vi "Tosca-Initialize Schedule State.vi"(0 "Tosca":refnum<class "Parameters.lvclass">, 11 "error in (no error)":errorcluster, 12 "Analysis In":T2, 13 "Controls":T1) -> (2 "Blocks":i32, 4 "Tosca out":refnum<class "Parameters.lvclass">, 14 "Analysis Out":T2, 15 "error out":errorcluster)   [LabVIEW 2020]
uses:
  Typedefs/Tosca-Analysis State.ctl
  Typedefs/Tosca-Adaptation State.ctl
  Typedefs/Tosca-Adaptation Track State.ctl
  Typedefs/Tosca-Adaptation History Element.ctl
  Classes/Parameters/Histogram Data.ctl
  Classes/Parameters/Connect.ctl
  Typedefs/Tosca-Control Refs.ctl
  FSM Graph VIs/LV Source/FSM Editor/FSM Editor.xctl
  Classes/Parameters/Parameters.lvclass
  Classes/Parameters/Parameters.lvclass/Parameters.ctl
  Classes/Parameters/Read Schedule.vi
  Classes/Parameters/Read Schedule Mode.vi
  Classes/Parameters/Read Adapt.vi
  Classes/Parameters/Write Adapt.vi
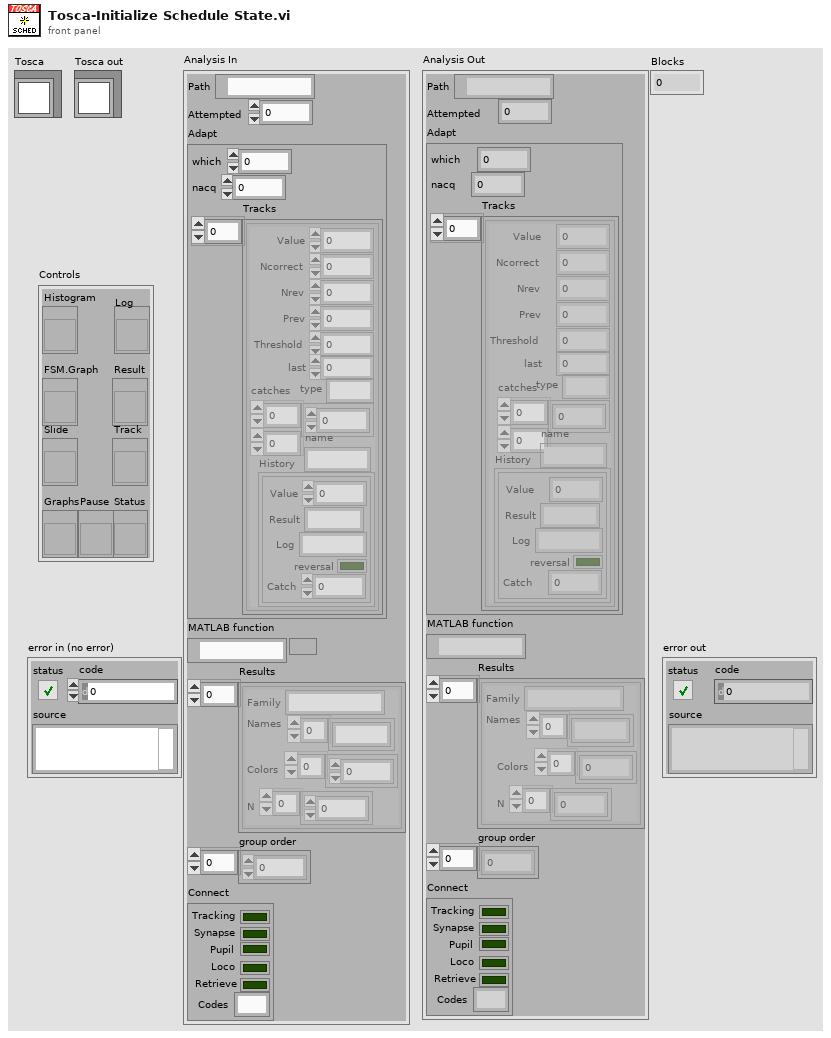
[diagram p1: front panel]
types:
  T1 = typedef "Tosca-Control Refs.ctl" = cluster{"FSM.Graph":refnum<vi>, "Slide":refnum<vi>, "Result":refnum<vi>, "Histogram":refnum<vi>, "Graphs":refnum<vi>, "Track":refnum<vi>, "Log":refnum<vi>, "Status":refnum<vi>, "Pause":refnum<vi>}
  T2 = typedef "Tosca-Analysis State.ctl" = cluster{"Path":path, "Attempted":i32, "Adapt":T3, "MATLAB function":path, "Results":T6[], "group order":i32[], "Connect":T7}
  T3 = typedef "Tosca-Adaptation State.ctl" = cluster{"which":i32, "nacq":i32, "Tracks":T4[]}
  T4 = typedef "Tosca-Adaptation Track State.ctl" = cluster{"Value":dbl, "Ncorrect":i32, "Nrev":i32, "Prev":dbl, "History":T5[], "Threshold":dbl, "last":i32, "type":string, "catches":dbl[][], "name":string}
  T5 = typedef "Tosca-Adaptation History Element.ctl" = cluster{"Value":dbl, "Result":string, "Log":string, "reversal":bool, "Catch":dbl}
  T6 = typedef "Parameters.lvclass/Histogram Data.ctl" = cluster{"Family":string, "Names":string[], "Colors":u32[], "N":i32[]}
  T7 = typedef "Parameters.lvclass/Connect.ctl" = cluster{"Tracking":bool, "Synapse":bool, "Pupil":bool, "Loco":bool, "Retrieve":bool, "Codes":string}
  T8 = typedef "Tosca-Schedule.ctl" = cluster{"Blocks":i32, "order":T9, "balance":bool, "Families":T10[]}
  T9 = typedef "Tosca-Sequence Order.ctl" = enum16{"Sequential", "Alternate", "Randomize", "Random group"}
  T10 = typedef "Tosca-Parameter Family.ctl" = cluster{"Name":string, "Number":i32, "Vars":T11[], "Mask":bool[][], "one each":bool}
  T11 = typedef "Tosca-Parameter Table Element.ctl" = cluster{"state":string, "chan":string, "param":string, "expr":string, "dim":T12, "value":dbl[]}
  T12 = typedef "Tosca-Parameter Dimension.ctl" = enum16{"Ind", "X", "Y"}
  T13 = typedef "Tosca-Schedule Mode.ctl" = enum16{"Seq", "CS+/CS-", "Adapt"}
  T14 = typedef "Tosca-Adapt.ctl" = cluster{"Switch after":i32, "Switch type":enum16{"Trials", "Reversals"}, "Tracks":T15[]}
  T15 = typedef "Tosca-Adaptive Track.ctl" = cluster{"state":string, "chan":string, "param":string, "Start":dbl, "Step":string, "Mode":enum16{"Add", "Multiply"}, "Pcatch":dbl, "Ndown":i32, "Nup":i32, "Nreverse":i32, "Min":dbl, "Max":dbl, "Catch":T16[], "do all catch":bool, "name":string, "Vars":T16[], "compute":T17, "of last":i32, "Step2":string, "after":i32}
  T16 = typedef "Tosca-Simple Variable.ctl" = cluster{"state":string, "chan":string, "param":string, "expr":string}
  T17 = typedef "Tosca-Adapt Threshold Metric.ctl" = enum16{"mean", "median"}
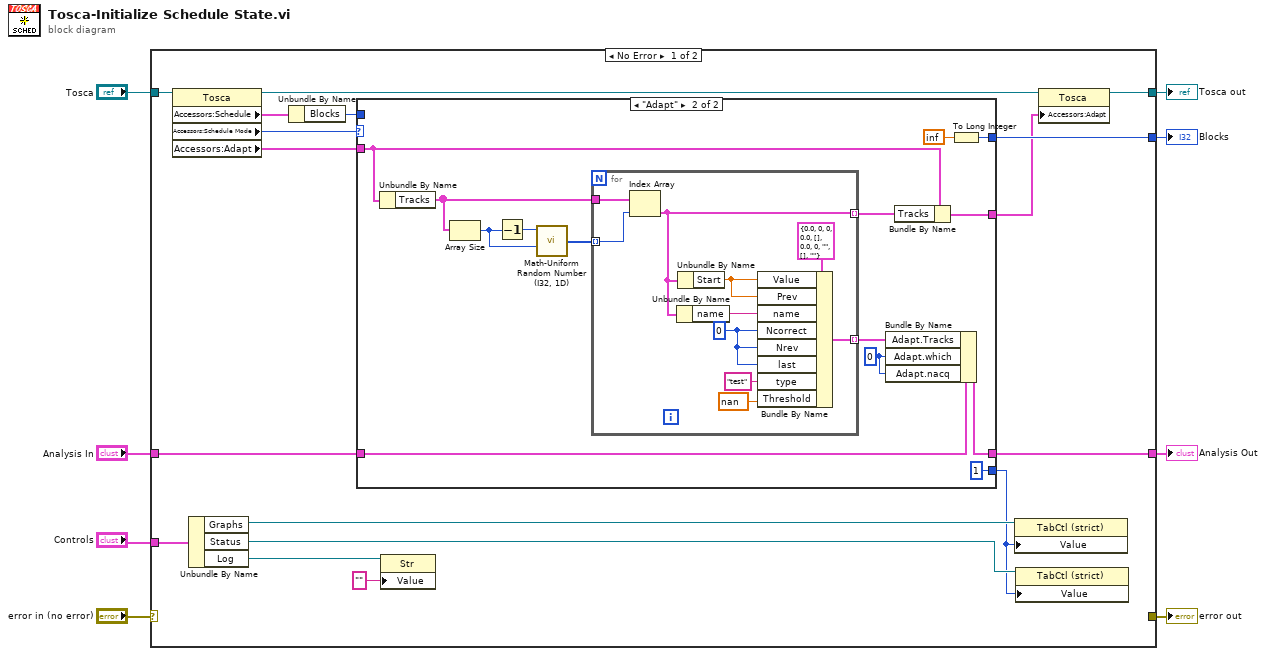
[diagram p0: block diagram]
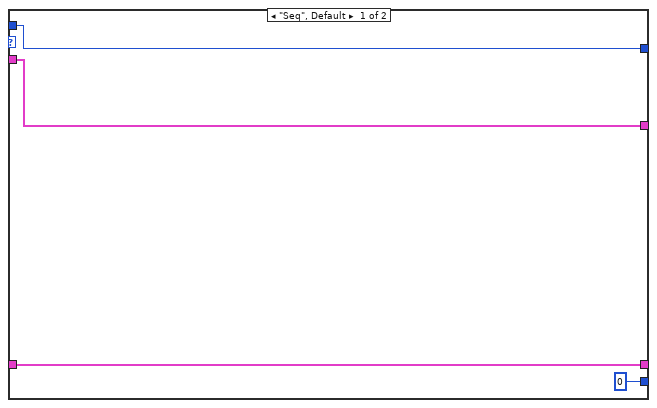
[diagram p2: hidden frame]
diagram:
  n1 = case shown="No Error" "error in (no error)" {
    selector: "error in (no error)" -> [_ w56]
    tunnel: [w24 _] -> w8
    tunnel: "Analysis In" -> [w23 w55]
    tunnel: [w22 w55] -> w6
    tunnel: [_ w56] -> w4
    tunnel: "Controls" -> [w21 _]
    tunnel: "Tosca" -> [w15 w54]
    tunnel: [w9 w54] -> w1
    frame No Error {
      n2 = property class="Tosca"(reference=w15) -> (reference out=w11:refnum<class "Parameters.lvclass">, "Accessors:Schedule"=w14:T8, "Accessors:Schedule Mode"=w13:T13, "Accessors:Adapt"=w12:T14)  [unwired: 1 in, 1 out]
      n3 = Unbundle By Name(w21) -> ("Graphs"=w20:refnum<vi>, "Status"=w19:refnum<vi>, "Log"=w18:refnum<vi>)
      n4 = Unbundle By Name(w14) -> ("Blocks"=w25:i32)
      n5 = case shown="\"Adapt\"" w13 {
        tunnel: w25 -> [w29 _]
        tunnel: [w29 w42] -> w24
        tunnel: w23 -> [w28 w40]
        tunnel: [w28 w39] -> w22
        tunnel: w12 -> [w26 w32]
        tunnel: [0 1] -> w16
        tunnel: [w26 w30] -> w10
        frame "Seq", Default {
        }
        frame "Adapt" {
          w37 = 0 ("Adapt.which")
          n6 = Unbundle By Name(w32) -> ("Tracks"=w36:T15[])
          n7 = Array Size(array=w36) -> (size(s)=w34:i32)
          n8 = Decrement(x=w34) -> (x-1=w35:i32)
          n9 = call "Math-Uniform Random Number (I32, 1D).vi"("N"=w34, "Ymax"=w35) -> ("Random Ints"=w33:i32[])  [unwired: 4 in]
          n10 = for {
            tunnel: w36 -> [w47]
            tunnel: [w50] -> w38 mode=indexing
            tunnel: w33 -> [w45] mode=indexing
            tunnel: [w44] -> w31 mode=indexing
            w53 = 0 ("Adapt.Ncorrect")
            n11 = Index Array(array=w47, index=w45) -> (element=w44:T15)
            n12 = Unbundle By Name(w44) -> ("name"=w46:string)
            n13 = Unbundle By Name(w44) -> ("Start"=w52:dbl)
            n14 = Bundle By Name(cluster=T4 {"Value"=0.0, "Ncorrect"=0, "Nrev"=0, "Prev"=0.0, "History"=[], "Threshold"=0.0, "last"=0, "type"="", "catches"=[], "name"=""} ("Adapt"), "Value"=w52, "Prev"=w52, "name"=w46, "Ncorrect"=w53, "Nrev"=w53, "last"=w53, "type"="test" ("last trial"), "Threshold"=nan) -> (w50:T4)
          }
          n15 = Bundle By Name(cluster=w40, "Adapt.Tracks"=w38, "Adapt.which"=w37, "Adapt.nacq"=w37) -> (w39:T2)
          n16 = Bundle By Name(cluster=w32, "Tracks"=w31) -> (w30:T14)
          n17 = To Long Integer(number=inf) -> (32bit integer=w42:i32)
        }
      }
      n18 = property class="Str"(reference=w18, "Value"="") -> ()  [unwired: 1 in, 2 out]
      n19 = property class="TabCtl (strict)"(reference=w20, "Value"=w16) -> ()  [unwired: 1 in, 2 out]
      n20 = property class="TabCtl (strict)"(reference=w19, "Value"=w16) -> ()  [unwired: 1 in, 2 out]
      n21 = property class="Tosca"(reference=w11, "Accessors:Adapt"=w10) -> (reference out=w9:refnum<class "Parameters.lvclass">)  [unwired: 1 in, 1 out]
    }
    frame Error {
    }
  }
  "error out" <- w4
  "Analysis Out" <- w6
  "Blocks" <- w8
  "Tosca out" <- w1
